vi "utility.TestDataAverage.vi"(7 "Igore times":u32, 9 "Test.Low.Limit":dbl, 10 "Test.High.Limit":dbl, 11 "TestData":dbl[](array[numeric])) -> (1 "Output TestData":dbl[](array[numeric]), 2 "OK?":bool, 3 "Average TestData":dbl)   [LabVIEW 2012, in "Lib_UEL.ATE.lvlib" / "Lib_App.lvlib"]
uses:
  Lib_App.lvlib
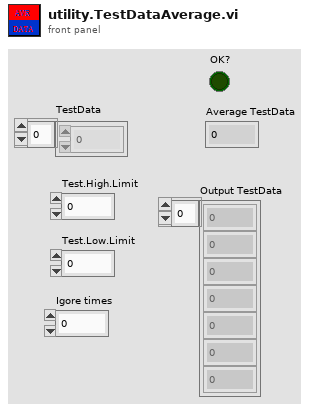
[diagram p1: front panel]
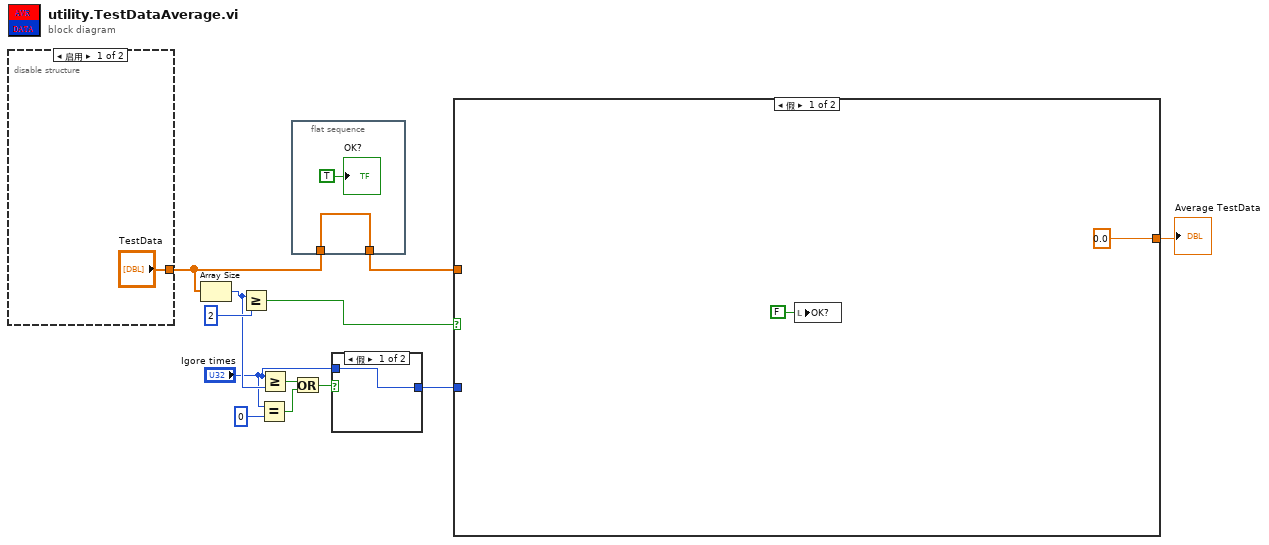
[diagram p0: block diagram]
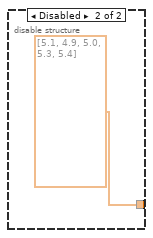
[diagram p2: hidden frame]
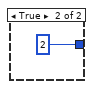
[diagram p3: hidden frame]
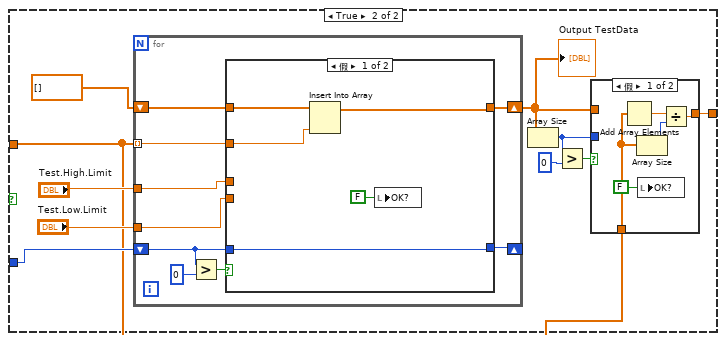
[diagram p4: hidden frame]
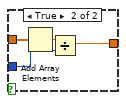
[diagram p5: hidden frame]
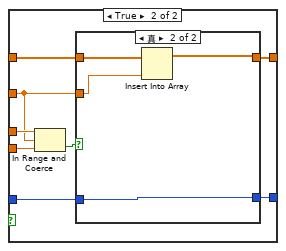
[diagram p6: hidden frame]
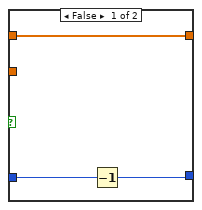
[diagram p7: hidden frame]
diagram:
  n1 = disable-structure shown="启用" {
    disable-tunnel: ["TestData" dbl[] [5.1, 4.9, 5.0, 5.3, 5.4] ("TestData")] -> w1
    frame Enabled {
    }
    frame Disabled {
    }
  }
  n2 = Array Size(array=w1) -> (size(s)=w10:i32)
  n3 = Greater Or Equal?(x=w10, y=2) -> (x >= y?=w11:bool)
  n4 = Equal?(x="Igore times", y=u32 0) -> (x = y?=w7:bool)
  n5 = Greater Or Equal?(x="Igore times", y=w10) -> (x >= y?=w8:bool)
  n6 = flat-sequence {
    tunnel: [w16] -> w2
    tunnel: w1 -> [w16]
    frame #0 {
      "OK?" <- TRUE ("OK?")
    }
  }
  n7 = Or(x=w8, y=w7) -> (x .or. y?=w6:bool)
  n8 = case shown="假" w6 {
    tunnel: [w17 u32 2 ("y")] -> w5
    tunnel: "Igore times" -> [w17 _]
    frame False {
    }
    frame True {
    }
  }
  n9 = case shown="假" w11 {
    tunnel: w2 -> [_ w21]
    tunnel: w5 -> [_ w27]
    tunnel: [0.0 w25] -> w3
    frame False {
      n10 = local write "OK?"(FALSE ("OK?")) -> ()
    }
    frame True {
      n11 = for {
        tunnel: w21 -> [w45] mode=indexing
        shift-right: [w44] -> w26
        shift-left: dbl[] [] -> [w46]
        tunnel: "Test.High.Limit" -> [w48]
        tunnel: "Test.Low.Limit" -> [w47]
        shift-right: [w43] -> _
        shift-left: w27 -> [w42]
        n12 = Greater?(x=w42, y=u32 0) -> (0:w40:bool)
        n13 = case shown="假" w40 {
          tunnel: w48 -> [_ w61]
          tunnel: w47 -> [_ w60]
          tunnel: w46 -> [w53 w59]
          tunnel: w45 -> [w52 w58]
          tunnel: [w51 w57] -> w44
          tunnel: [w50 w56] -> w43
          tunnel: w42 -> [w50 w55]
          frame False {
            n14 = Insert Into Array(array=w53, new element=w52) -> (w51:dbl[])  [unwired: 1 in]
            n15 = local write "OK?"(FALSE ("OK?")) -> ()
          }
          frame True {
            n16 = In Range and Coerce(upper limit=w61, x=w58, lower limit=w60) -> (In Range?=w54:bool)  [unwired: 1 out]
            n17 = case shown="真" w54 {
              tunnel: w59 -> [w64 w68]
              tunnel: w58 -> [_ w67]
              tunnel: [w64 w66] -> w57
              tunnel: w55 -> [w63 w65]
              tunnel: [w62 w65] -> w56
              frame False {
                n18 = Decrement(x=w63) -> (x-1=w62:u32)
              }
              frame True {
                n19 = Insert Into Array(array=w68, new element=w67) -> (w66:dbl[])  [unwired: 1 in]
              }
            }
          }
        }
      }
      "Output TestData" <- w26
      n20 = Array Size(array=w26) -> (size(s)=w24:i32)
      n21 = Greater?(x=w24, y=0) -> (0:w22:bool)
      n22 = case shown="假" w22 {
        tunnel: w26 -> [_ w39]
        tunnel: [w34 w37] -> w25
        tunnel: w24 -> [_ w36]
        tunnel: w21 -> [w35 _]
        frame False {
          n23 = Add Array Elements(numeric array=w35) -> (sum=w33:dbl)
          n24 = Array Size(array=w35) -> (size(s)=w32:i32)
          n25 = local write "OK?"(FALSE ("OK?")) -> ()
          n26 = Divide(x=w33, y=w32) -> (x/y=w34:dbl)
        }
        frame True {
          n27 = Add Array Elements(numeric array=w39) -> (sum=w38:dbl)
          n28 = Divide(x=w38, y=w36) -> (x/y=w37:dbl)
        }
      }
    }
  }
  "Average TestData" <- w3
